vi "Launch User Selection.vi"(8 "error in (no error)":errorcluster, 11 "ImageLoad in":refnum<class "ImageLoad.lvclass">) -> (0 "error out":errorcluster, 1 "Success?(True)":bool, 3 "ImageLoad out":refnum<class "ImageLoad.lvclass">)   [LabVIEW 2015, in "ImageLoad.lvclass"]
uses:
  ImageLoad.lvclass
  <vilib>/Utility/miscctls.llb/LVBrowseOptionsTypeDef.ctl
  ImageLoad.lvclass/ImageLoad.ctl
panel:
  in  "TargetFile Options":T1={"Prompt"="", "Match Pattern"="", "Mode"=enum."existing dir", "Start Path"=path "", "Pattern Label"="select Target Directory", "Button Text"=""}
  in  "SourceFile Options":T1={"Prompt"="", "Match Pattern"="", "Mode"=enum."existing dir", "Start Path"=path "", "Pattern Label"="select Source Directory", "Button Text"=""}
  in  "Target File Folder":path
  in  "Source File":path
  in  "Cancel":bool
  in  "Sure":bool
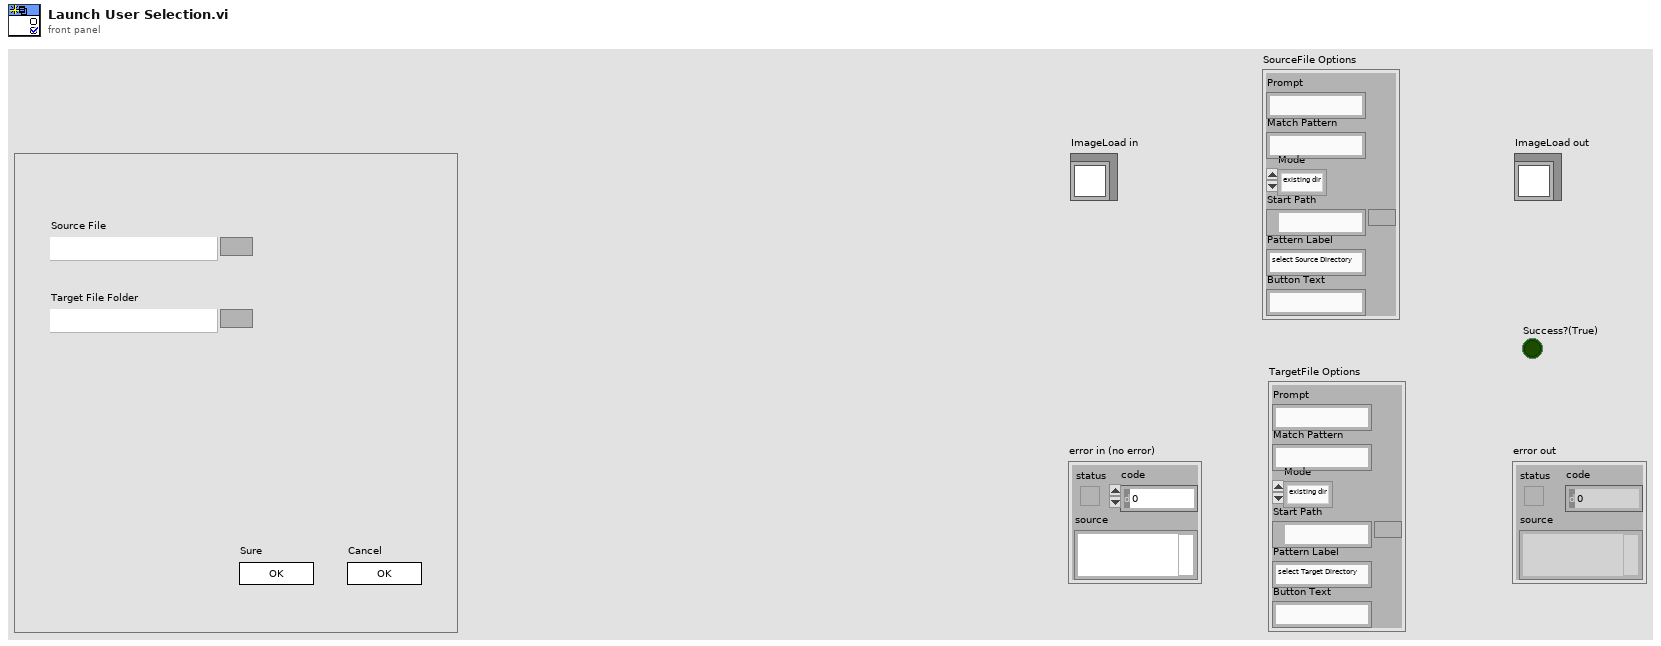
[diagram p1: front panel]
types:
  T1 = typedef "LVBrowseOptionsTypeDef.ctl" = cluster{"Prompt":string, "Match Pattern":string, "Mode":enum32{"existing file", "new file", "new or existing file", "existing dir", "new dir", "new or existing dir", "existing file (use LLBs)", "new file (use LLBs)", "new or existing file (use LLBs)", "new or existing file or directory (use LLBs)", "existing dir (use LLBs)", "new dir (use LLBs)", "new or existing dir (use LLBs)", "existing file or dir", "new file or dir", "new or existing file or dir", "existing file or dir (use LLBs)", "new file or dir (use LLBs)"}, "Start Path":path, "Pattern Label":string, "Button Text":string}
  T2 = enum32{"Invalid", "Standard", "Closed", "Hidden", "Minimized", "Maximized"}
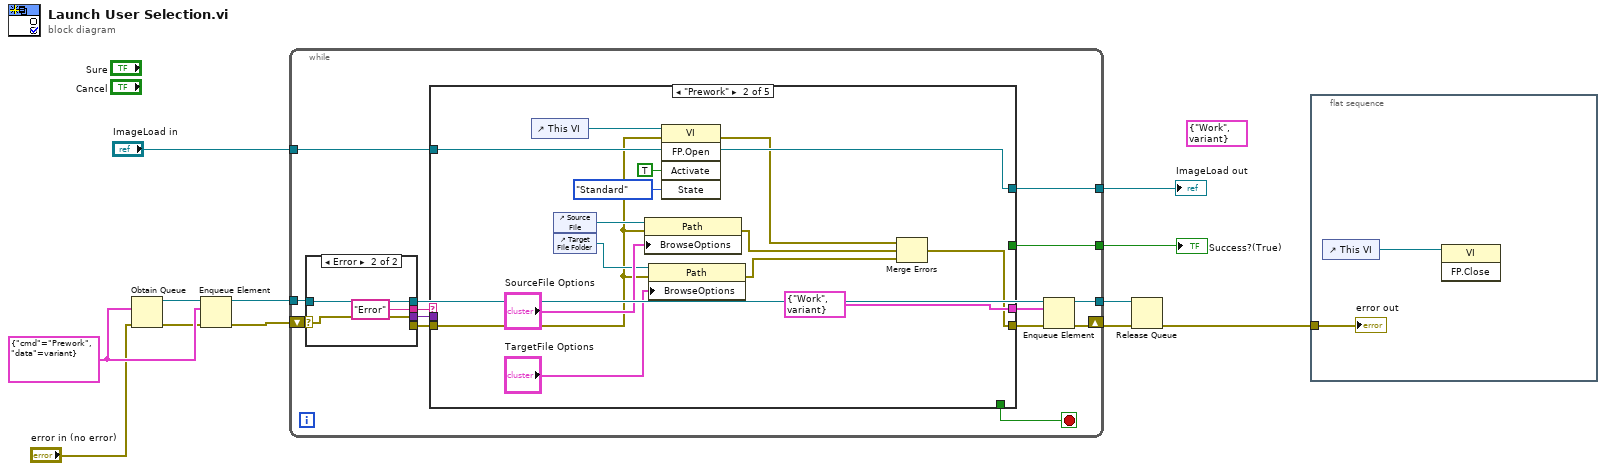
[diagram p0: block diagram]
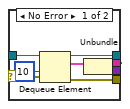
[diagram p2: hidden frame]
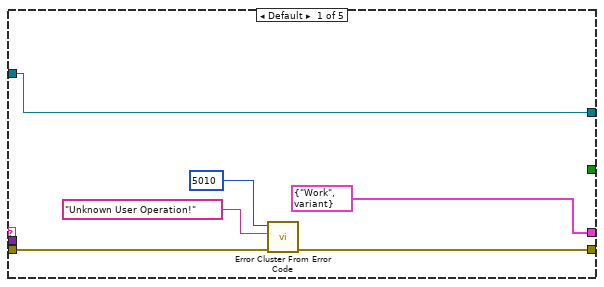
[diagram p3: hidden frame]
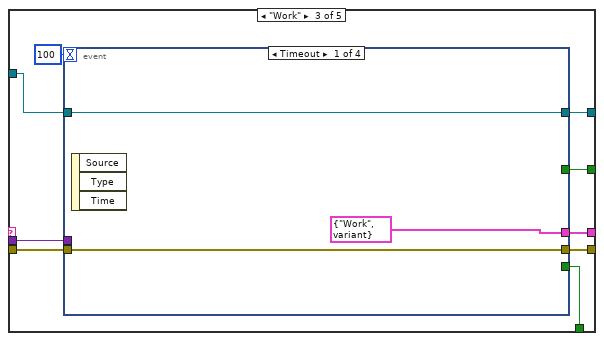
[diagram p4: hidden frame]
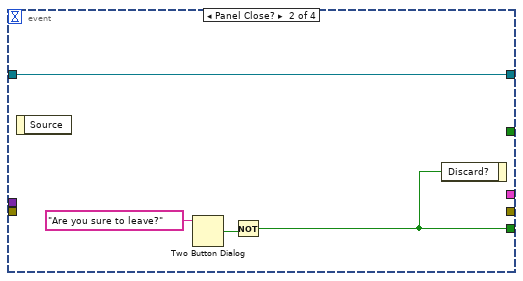
[diagram p5: hidden frame]
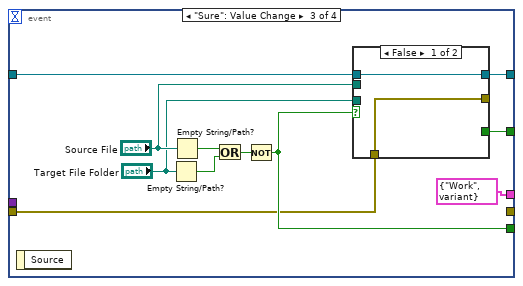
[diagram p6: hidden frame]
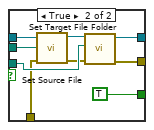
[diagram p7: hidden frame]
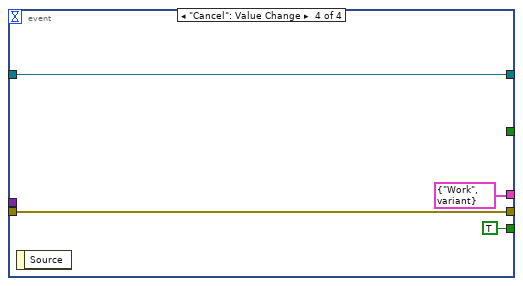
[diagram p8: hidden frame]
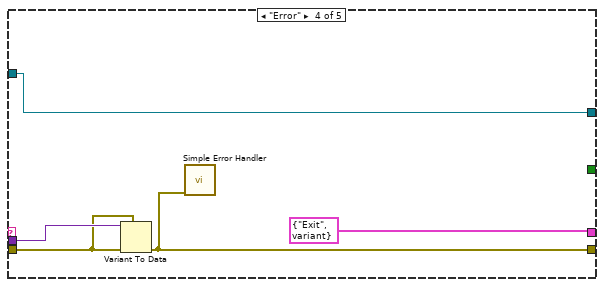
[diagram p9: hidden frame]
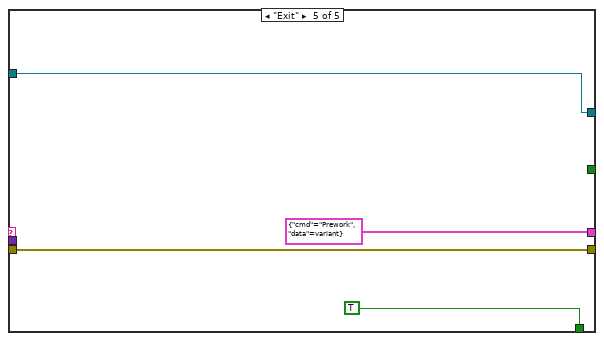
[diagram p10: hidden frame]
diagram:
  (unwired) cluster{"cmd":string, "data":variant} {"cmd"="Work", "data"=variant}
  w10 = cluster{"cmd":string, "data":variant} {"cmd"="Prework", "data"=variant}
  n1 = Obtain Queue(element data type=w10, error in (no error)="error in (no error)") -> (queue out=w6:refnum<queue>, error out=w7:errorcluster)  [unwired: 3 in, 1 out]
  n2 = Enqueue Element(queue=w6, element=w10, error in (no error)=w7) -> (queue out=w8:refnum<queue>, error out=w9:errorcluster)  [unwired: 1 in, 1 out]
  n3 = while {
    tunnel: w8 -> [w25]
    tunnel: [w17] -> w11
    shift-right: [w16] -> w12
    shift-left: w9 -> [w26]
    tunnel: "ImageLoad in" -> [w15]
    tunnel: [w14] -> w3
    tunnel: [w13] -> w2
    stop <- w18 stop-if-true
    n4 = case shown="Error" w26 {
      selector: w26 -> [w33 w36]
      tunnel: w25 -> [w34 w37]
      tunnel: [w31 w37] -> w23
      tunnel: [w30 _] -> w21
      tunnel: [w28 "Error" ("cmd")] -> w22
      tunnel: [w27 w36] -> w24
      frame No Error {
        n5 = Dequeue Element(queue=w34, timeout in ms (-1)=10, error in (no error)=w33) -> (queue out=w31:refnum<queue>, element=w29:cluster{"cmd":string, "data":variant}, error out=w30:errorcluster)  [unwired: 1 out]
        n6 = Unbundle(w29) -> ("cmd"=w28:string, "data"=w27:variant)
      }
      frame Error {
      }
    }
    n7 = case shown="\"Prework\"" w22 {
      tunnel: w24 -> [_ _ w66 w104 _]
      tunnel: w21 -> [w40 w45 w65 w103 w108]
      tunnel: [cluster{"cmd":string, "data":variant} {"cmd"="Work", "data"=variant} cluster{"cmd":string, "data":variant} {"cmd"="Work", "data"=variant} w63 cluster{"cmd":string, "data":variant} {"cmd"="Exit", "data"=variant} cluster{"cmd":string, "data":variant} {"cmd"="Prework", "data"=variant}] -> w20
      tunnel: [w41 w50 w62 w101 w108] -> w19
      tunnel: [_ _ w61 _ TRUE] -> w18
      tunnel: w15 -> [w38 w49 w60 w100 w105]
      tunnel: [w38 w49 w59 w100 w105] -> w14
      tunnel: [_ _ w58 _ _] -> w13
      frame Default {
        n8 = call <vilib>:"Error Cluster From Error Code.vi"("error in (no error)"=w40, "error message (\"\")"="Unknown User Operation!" ("error message (\"\")"), "error code (0)"=5010) -> ("error out"=w41:errorcluster)  [unwired: 6 in]
      }
      frame "Prework" {
        n9 = control-ref of="This VI"() -> (w48:refnum<vi>)
        n10 = control-ref of="Source File"() -> (w56:refnum<vi>)
        n11 = control-ref of="Target File Folder"() -> (w54:refnum<vi>)
        n12 = property class="Path"(reference=w56, error in=w45, "BrowseOptions"="SourceFile Options") -> (error out=w52:errorcluster)  [unwired: 1 out]
        n13 = property class="Path"(reference=w54, error in=w45, "BrowseOptions"="TargetFile Options") -> (error out=w51:errorcluster)  [unwired: 1 out]
        n14 = invoke class="VI" method="FP.Open"(reference=w48, error in=w45, "Activate"=TRUE ("Activate?"), "State"=T2."Standard") -> (error out=w44:errorcluster)  [unwired: 1 in, 4 out]
        n15 = Merge Errors(w44, w52, w51) -> (w50:errorcluster)
      }
      frame "Work" {
        n16 = event shown="[0] Timeout" {
          selector: _ -> [_ _ _ _]
          dyn-events: _ -> [_ _ _ _]
          timeout: 100 -> [_ _ _ _]
          tunnel: w66 -> [_ _ _ _]
          tunnel: w65 -> [w68 _ w76 w98]
          tunnel: [cluster{"cmd":string, "data":variant} {"cmd"="Work", "data"=variant} _ cluster{"cmd":string, "data":variant} {"cmd"="Work", "data"=variant} cluster{"cmd":string, "data":variant} {"cmd"="Work", "data"=variant}] -> w63
          tunnel: [w68 _ _ w98] -> w62
          tunnel: [_ w71 w80 TRUE] -> w61
          tunnel: w60 -> [w67 w70 w79 w99]
          tunnel: [w67 w70 w75 w99] -> w59
          tunnel: [_ _ w74 _] -> w58
          event Timeout {
            n17 = event-data() -> ()  [unwired: 1 in, 3 out]
          }
          event Panel Close? {
            n18 = event-data() -> ()  [unwired: 1 in, 1 out]
            n19 = Two Button Dialog(message="Are you sure to leave?") -> (T button?=w72:bool)  [unwired: 2 in]
            n20 = Not(x=w72) -> (.not. x?=w71:bool)
            n21 = event-data("Discard?"=w71) -> ()  [unwired: 1 in, 1 out]
          }
          event "Sure": Value Change {
            n22 = event-data() -> ()  [unwired: 1 in, 1 out]
            n23 = Empty String/Path?(string/path="Target File Folder") -> (empty?=w83:bool)
            n24 = Empty String/Path?(string/path="Source File") -> (empty?=w84:bool)
            n25 = Or(x=w84, y=w83) -> (x .or. y?=w81:bool)
            n26 = Not(x=w81) -> (.not. x?=w80:bool)
            n27 = case shown="False" w80 {
              tunnel: w79 -> [w86 w95]
              tunnel: "Source File" -> [_ w94]
              tunnel: "Target File Folder" -> [_ w93]
              tunnel: w76 -> [w85 w91]
              tunnel: [w86 w89] -> w75
              tunnel: [w85 w88] -> _
              tunnel: [_ TRUE] -> w74
              frame False {
              }
              frame True {
                n28 = call "Set Source File.vi"("error in (no error)"=w91, "Source File"=w94, "ImageLoad in"=w95) -> ("error out"=w90:errorcluster, "ImageLoad out"=w92:refnum<class "ImageLoad.lvclass">)  [unwired: 7 in]
                n29 = call "Set Target File Folder.vi"("error in (no error)"=w90, "Target File Folder"=w93, "ImageLoad in"=w92) -> ("error out"=w88:errorcluster, "ImageLoad out"=w89:refnum<class "ImageLoad.lvclass">)  [unwired: 7 in]
              }
            }
          }
          event "Cancel": Value Change {
            n30 = event-data() -> ()  [unwired: 1 in, 1 out]
          }
        }
      }
      frame "Error" {
        n31 = Variant To Data(error in=w103, type=w103, Variant=w104) -> (error out=w101:errorcluster)  [unwired: 1 out]
        n32 = call <vilib>:"Simple Error Handler.vi"("error in (no error)"=w101) -> ()  [unwired: 4 in, 5 out]
      }
      frame "Exit" {
      }
    }
    n33 = Enqueue Element(queue=w23, element=w20, error in (no error)=w19) -> (queue out=w17:refnum<queue>, error out=w16:errorcluster)  [unwired: 1 in, 1 out]
  }
  "ImageLoad out" <- w3
  "Success?(True)" <- w2
  n34 = Release Queue(queue=w11, error in (no error)=w12) -> (error out=w1:errorcluster)  [unwired: 1 in, 2 out]
  n35 = flat-sequence {
    tunnel: w1 -> [w109]
    frame #0 {
      n36 = control-ref of="This VI"() -> (w110:refnum<vi>)
      n37 = invoke class="VI" method="FP.Close"(reference=w110) -> ()  [unwired: 2 in, 3 out]
      "error out" <- w109
    }
  }
